vi "PI Dialog Number Pad.vi"(7 "Prompt":string, 8 "error in (no error)":errorcluster, 9 "Limit Text":string, 10 "Use Decimal? (f)":bool, 11 "Number (\"0.0\")":string="0.0") -> (0 "error out":errorcluster, 1 "Number":dbl, 2 "Cancelled?":bool, 3 "Number":string)   [LabVIEW 2011]
doc: "This Utility vi operates as a limited keyboard input for the BaseStAR user. All keys are upper case, no shift (or control, alt, etc.) keys are offered. There are 36 keys arranged as the standard 'QWERTY' type keyboard with numbers along the top row. Two additional keys are given as 'SPACE' and 'BACKSPACE'. Finally, there is a 'CLEAR' button along the menubar. Contents of the string indicator are passed out of the vi when the user presses the 'OK' button on the menubar.\n\nGlobals Used:\n* Root\n* Panel Geometry\n* Sound\n\nProgramming Notes:\ni) Depending upon Sound global, this VI will play a sound for each key press. The sound played is hard-coded as a .wav audio file normally found in the file 'Sound\\keyclick.wav'.\n\nii) The keyboard's Nominal Repeat Rate will increase to the Maximum Repeat Rate after a particular key is held down for a preset number of consecutive times. All three of these parameters are hard-coded."
uses:
  Keystroke.ctl
panel:
  in  "Buffer":string
  in  ".":bool caption="Add Field"
  in  "0":bool caption="Add Field"
  in  "Plus Minus":bool caption="Add Field"
  in  "3":bool caption="Add Field"
  in  "2":bool caption="Add Field"
  in  "1":bool caption="Add Field"
  in  "6":bool caption="Add Field"
  in  "5":bool caption="Add Field"
  in  "4":bool caption="Add Field"
  in  "9":bool caption="Add Field"
  in  "8":bool caption="Add Field"
  in  "7":bool caption="Add Field"
  in  "Clear":bool caption="Add Field"
  in  "Cancel":bool caption="Add Field"
  in  "OK":bool caption="Add Field"
  # "NUMBER PAD I/O"
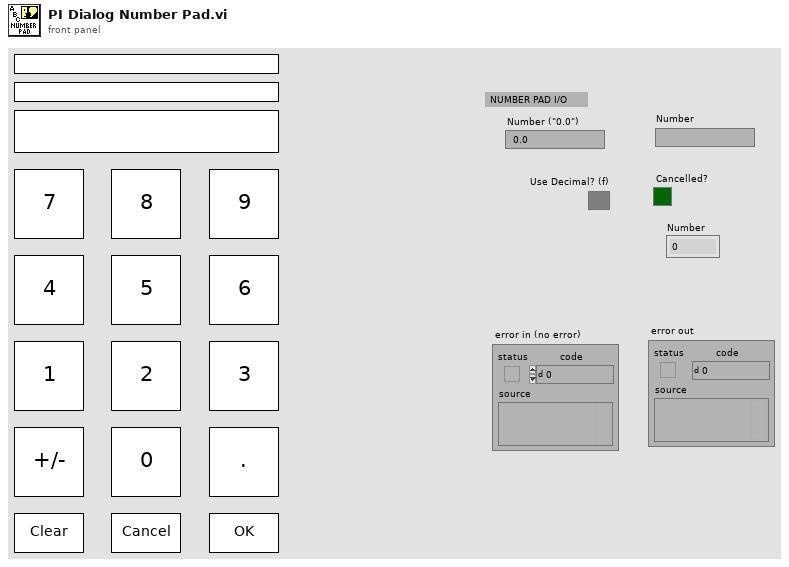
[diagram p1: front panel]
types:
  T1 = cluster{"left":i16, "top":i16, "right":i16, "bottom":i16}
  T2 = enum8{"Enabled", "Disabled", "Disabled and Grayed Out"}
  T3 = typedef "Keystroke.ctl" = enum16{"None", "CTRL+ALT+A", "CTRL+ALT+F", "CTRL+ALT+L", "CTRL+ALT+M", "CTRL+ALT+P", "CTRL+ALT+R"}
  T4 = cluster{"Selection Start":u32, "Selection End":u32}
  T5 = typedef "eventvkey.ctl" = enum16{"ASCII", "Enter", "Return", "Shift", "Ctrl", "Alt", "Cmd", "Opt", "Caps", "NumLock", "Clear", "Break", "Up", "Down", "Left", "Right", "Insert", "Delete", "Home", "End", "PageUp", "PageDown", "Escape", "Help", "Pause", "ScrollLock", "F1", "F2", "F3", "F4", "F5", "F6", "F7", "F8", "F9", "F10", "F11", "F12", "F13", "F14", "F15", "F16", "F17", "F18", "F19", "F20", "F21", "F22", "F23", "F24", "Play", "VolumeUp", "VolumeDown", "Mute", "Two Byte Char"}
  T6 = cluster{"Shift":bool, "Ctrl":bool, "Alt":bool, "Cmd":bool, "Opt":bool}
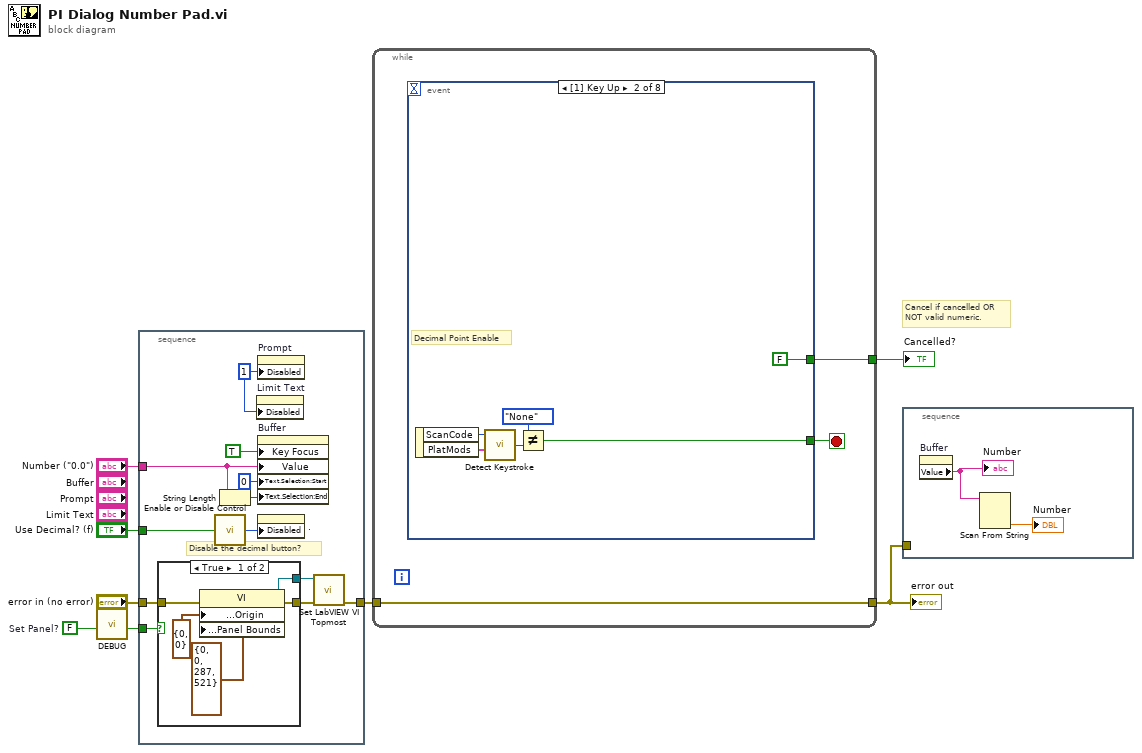
[diagram p0: block diagram]
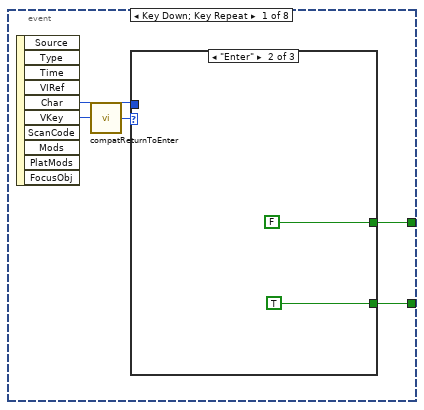
[diagram p2: hidden frame]
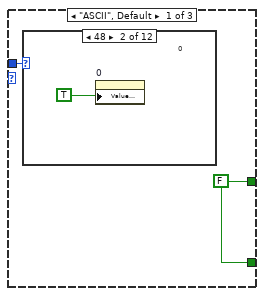
[diagram p3: hidden frame]
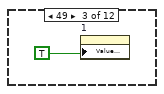
[diagram p5: hidden frame]
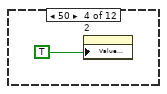
[diagram p6: hidden frame]
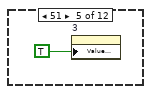
[diagram p7: hidden frame]
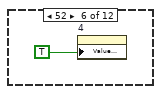
[diagram p8: hidden frame]
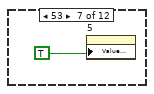
[diagram p9: hidden frame]
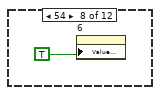
[diagram p10: hidden frame]
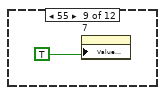
[diagram p11: hidden frame]
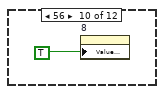
[diagram p12: hidden frame]
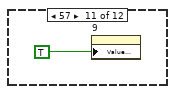
[diagram p13: hidden frame]
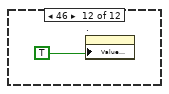
[diagram p14: hidden frame]
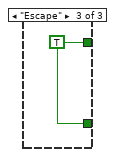
[diagram p15: hidden frame]
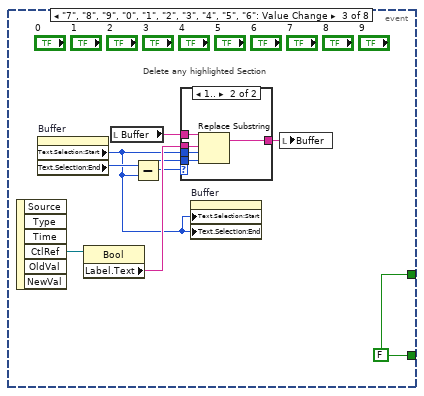
[diagram p16: hidden frame]
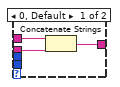
[diagram p17: hidden frame]
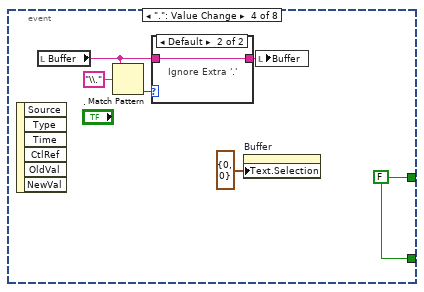
[diagram p18: hidden frame]
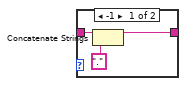
[diagram p19: hidden frame]
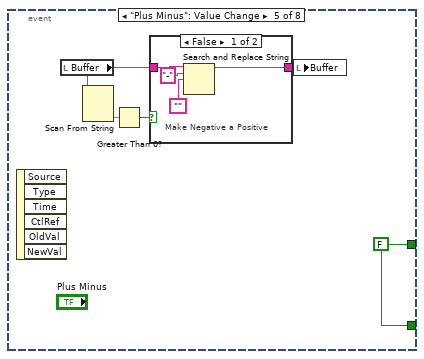
[diagram p20: hidden frame]
diagram:
  w2 = FALSE  # Set Panel?
  # "Cancel if cancelled OR\nNOT valid numeric."
  n1 = call "DEBUG.vi"("Dev DEBUG? (f)"=w2) -> ("DEBUG?"=w1:bool)  [unwired: 1 in, 5 out]
  n2 = stacked-sequence {
    tunnel: [w16] -> w8
    tunnel: "error in (no error)" -> [w15]
    tunnel: "Use Decimal? (f)" -> [w14]
    tunnel: "Number (\"0.0\")" -> [w11]
    tunnel: w1 -> [w9]
    frame #0 {
      w19 = u8 1 ("Disabled")
      # "Disable the decimal button?"
      n3 = case shown="True" w9 {
        tunnel: [w25 w29] -> w18
        tunnel: [w24 w28] -> w17
        tunnel: w15 -> [w23 w27]
        frame True {
          n4 = property class="VI"(error in=w23, "Front Panel Window:Origin"=cluster{"Horizontal":i16, "Vertical":i16} {"Horizontal"=0, "Vertical"=0}, "Front Panel Window:Panel Bounds"=T1 {"left"=0, "top"=0, "right"=287, "bottom"=521}) -> (reference out=w25:refnum<vi>, error out=w24:errorcluster)  [unwired: 1 in]
        }
        frame False {
          n5 = property class="VI"(error in=w27, "Front Panel Window:Open"=TRUE) -> (reference out=w29:refnum<vi>, error out=w28:errorcluster)  [unwired: 1 in]
        }
      }
      n6 = call "Enable or Disable Control.vi"("Enable? (T)"=w14) -> ("Enable\\Disable"=w20:T2)
      n7 = String Length(string=w11) -> (length=w12:i32)
      n8 = property on="Limit Text" class="Str"("Disabled"=w19) -> ()  [unwired: 2 in, 2 out]
      n9 = property on="Prompt" class="Str"("Disabled"=w19) -> ()  [unwired: 2 in, 2 out]
      n10 = property on="Buffer" class="Str"("Key Focus"=TRUE, "Value"=w11, "Text.Selection:Start"=u8 0 ("Disabled"), "Text.Selection:End"=w12) -> ()  [unwired: 2 in, 2 out]
      n11 = property on="." class="Bool"("Disabled"=w20) -> ()  [unwired: 2 in, 2 out]
      n12 = call "Set LabVIEW VI Topmost.vi"("error in (no error)"=w17, "VI Refnum (null)"=w18) -> ("error out"=w16:errorcluster)  [unwired: 7 in, 2 out]
    }
  }
  n13 = while {
    tunnel: [w32] -> w6
    tunnel: w8 -> [w32]
    tunnel: [w30] -> w7
    stop <- w31 stop-if-true
    # "Decimal Point Enable"
    n14 = event shown="[1] Key Up" {
      selector: _ -> [_ _ _ _ _ _ _ _]
      dyn-events: _ -> [_ _ _ _ _ _ _ _]
      timeout: _ -> [_ _ _ _ _ _ _ _]
      tunnel: [w35 w54 w66 w80 w88 FALSE TRUE TRUE] -> w31
      tunnel: [w34 FALSE ("Cancel") w66 w80 w88 FALSE ("Cancel") "Cancel" FALSE ("Cancel")] -> w30
      event Key Down; Key Repeat {
        n15 = event-data() -> ("Char"=w37:i16, "VKey"=w33:T5)  [unwired: 9 out]
        n16 = call <vilib>:"compatReturnToEnter.vi"("VKey"=w33) -> ("VKey"=w36:T5)
        n17 = case shown="\"Enter\"" w36 {
          tunnel: w37 -> [w39 _ _]
          tunnel: [w38 TRUE w53] -> w35
          tunnel: [w38 FALSE w53] -> w34
          frame "ASCII", Default {
            w38 = FALSE
            n18 = case shown="48" w39 {
              frame Default {
              }
              frame 48 {
                # "0"
                n19 = property on="0" class="Bool"("Value (Signaling)"=TRUE) -> ()  [unwired: 2 in, 2 out]
              }
              frame 49 {
                n20 = property on="1" class="Bool"("Value (Signaling)"=TRUE) -> ()  [unwired: 2 in, 2 out]
              }
              frame 50 {
                n21 = property on="2" class="Bool"("Value (Signaling)"=TRUE) -> ()  [unwired: 2 in, 2 out]
              }
              frame 51 {
                n22 = property on="3" class="Bool"("Value (Signaling)"=TRUE) -> ()  [unwired: 2 in, 2 out]
              }
              frame 52 {
                n23 = property on="4" class="Bool"("Value (Signaling)"=TRUE) -> ()  [unwired: 2 in, 2 out]
              }
              frame 53 {
                n24 = property on="5" class="Bool"("Value (Signaling)"=TRUE) -> ()  [unwired: 2 in, 2 out]
              }
              frame 54 {
                n25 = property on="6" class="Bool"("Value (Signaling)"=TRUE) -> ()  [unwired: 2 in, 2 out]
              }
              frame 55 {
                n26 = property on="7" class="Bool"("Value (Signaling)"=TRUE) -> ()  [unwired: 2 in, 2 out]
              }
              frame 56 {
                n27 = property on="8" class="Bool"("Value (Signaling)"=TRUE) -> ()  [unwired: 2 in, 2 out]
              }
              frame 57 {
                n28 = property on="9" class="Bool"("Value (Signaling)"=TRUE) -> ()  [unwired: 2 in, 2 out]
              }
              frame 46 {
                n29 = property on="." class="Bool"("Value (Signaling)"=TRUE) -> ()  [unwired: 2 in, 2 out]
              }
            }
          }
          frame "Enter" {
          }
          frame "Escape" {
            w53 = TRUE
          }
        }
      }
      event Key Up {
        n30 = event-data() -> ("ScanCode"=w59:i16, "PlatMods"=w58:T6)  [unwired: 1 out]
        n31 = call "Detect Keystroke.vi"("PlatMods"=w58, "ScanCode"=w59) -> ("Keystroke"=w55:T3)  [unwired: 4 out]
        n32 = Not Equal?(x=Keystroke."None", y=w55) -> (x != y?=w54:bool)
      }
      event "7", "8", "9", "0", "1", "2", "3", "4", "5", "6": Value Change {
        w66 = FALSE
        # "Delete any highlighted Section"
        n33 = event-data() -> ("CtlRef"=w67:refnum<vi>)  [unwired: 6 out]
        n34 = property on="Buffer" class="Str"() -> ("Text.Selection:Start"=w63:u32, "Text.Selection:End"=w64:u32)  [unwired: 2 in, 2 out]
        n35 = property class="Bool"(reference=w67) -> ("Label.Text"=w65:string)  [unwired: 1 in, 2 out]
        n36 = local read "Buffer"() -> (w61:string)
        n37 = Subtract(x=w64, y=w63) -> (x-y=w62:u32)
        n38 = case shown="1.." w62 {
          tunnel: w65 -> [w69 w75]
          tunnel: [w68 w74] -> w60
          tunnel: w61 -> [w70 w73]
          tunnel: w63 -> [_ w72]
          tunnel: w62 -> [_ w71]
          frame 0, Default {
            n39 = Concatenate Strings(w70, w69) -> (w68:string)
          }
          frame 1.. {
            n40 = Replace Substring(2:w71, 3:w72, 4:w75, 5:w73) -> (1:w74:string)  [unwired: 1 out]
          }
        }
        n41 = property on="Buffer" class="Str"("Text.Selection:Start"=w63, "Text.Selection:End"=w63) -> ()  [unwired: 2 in, 2 out]
        n42 = local write "Buffer"(w60) -> ()
      }
      event ".": Value Change {
        w80 = FALSE ("Cancel")
        n43 = event-data() -> ()  [unwired: 7 out]
        n44 = local read "Buffer"() -> (w77:string)
        n45 = Match Pattern(string=w77, regular expression="\\.") -> (offset past match=w79:i32)  [unwired: 4 out]
        n46 = case shown="Default" w79 {
          tunnel: w77 -> [w84 w85]
          tunnel: [w83 w85] -> w76
          frame -1 {
            n47 = Concatenate Strings(w84, ".") -> (w83:string)
          }
          frame Default {
            # "Ignore Extra '.'"
          }
        }
        n48 = property on="Buffer" class="Str"("Text.Selection"=T4 {"Selection Start"=0, "Selection End"=0}) -> ()  [unwired: 2 in, 2 out]
        n49 = local write "Buffer"(w76) -> ()
      }
      event "Plus Minus": Value Change {
        w88 = FALSE ("Cancel")
        n50 = event-data() -> ()  [unwired: 7 out]
        n51 = local read "Buffer"() -> (w87:string)
        n52 = Scan From String(input string=w87) -> (output 1=w90:dbl)  [unwired: 3 in, 4 out]
        n53 = Greater Than 0?(x=w90) -> (x > 0?=w89:bool)
        n54 = case shown="False" w89 {
          tunnel: w87 -> [w94 w96]
          tunnel: [w91 w95] -> w86
          frame False {
            # "Make Negative a Positive"
            n55 = Search and Replace String(input string=w94, search string="-", replace string="") -> (result string=w91:string)  [unwired: 1 in, 7 out]
          }
          frame True {
            # "Make Positive a Negative"
            n56 = Concatenate Strings("-", w96) -> (w95:string)
          }
        }
        n57 = local write "Buffer"(w86) -> ()
      }
      event "Clear": Value Change {
        n58 = event-data() -> ()  [unwired: 7 out]
        n59 = local write "Buffer"("") -> ()
      }
      event "Cancel": Value Change {
        n60 = event-data() -> ()  [unwired: 7 out]
      }
      event "OK": Value Change {
        n61 = event-data() -> ()  [unwired: 7 out]
      }
    }
  }
  "Cancelled?" <- w7
  "error out" <- w6
  n62 = stacked-sequence {
    tunnel: w6 -> [_]
    frame #0 {
      n63 = property on="Buffer" class="Str"() -> ("Value"=w105:string)  [unwired: 2 in, 2 out]
      "Number" <- w105
      n64 = Scan From String(input string=w105) -> (output 1=→"Number":dbl)  [unwired: 3 in, 4 out]
    }
  }
